vi "Acquire Connection.vi"(4 "error in (no error)":errorcluster, 7 "Connection String":string) -> (0 "error out":errorcluster, 2 "ADO Version":string, 3 "Connection":refnum<k7>)   [LabVIEW 2020, in "ADO Database Drivers.lvlib"]
uses:
  ADO Database Drivers.lvlib
panel:
  in  "?":refnum<k7>
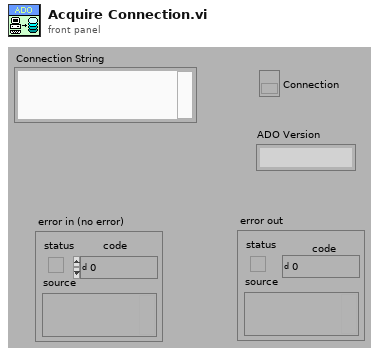
[diagram p1: front panel]
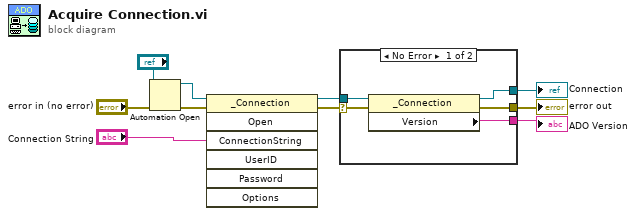
[diagram p0: block diagram]
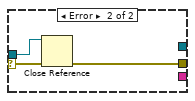
[diagram p2: hidden frame]
diagram:
  n1 = Automation Open(error in (no error)="error in (no error)", Automation Refnum="?") -> (Automation Refnum=w6:refnum<k7>, error out=w7:errorcluster)  [unwired: 2 in]
  n2 = invoke class="_Connection" method="Open"(reference=w6, error in=w7, "ConnectionString"="Connection String") -> (reference out=w4:refnum<k7>, error out=w5:errorcluster)  [unwired: 4 in, 5 out]
  n3 = case shown="No Error" w5 {
    selector: w5 -> [w15 w17]
    tunnel: w4 -> [w14 w18]
    tunnel: [w12 w16] -> w3
    tunnel: [w13 _] -> w2
    tunnel: [w11 _] -> w1
    frame No Error {
      n4 = property class="_Connection"(reference=w14, error in=w15) -> (reference out=w13:refnum<k7>, error out=w12:errorcluster, "Version"=w11:string)
    }
    frame Error {
      n5 = Close Reference(reference=w18, error in (no error)=w17) -> (error out=w16:errorcluster)
    }
  }
  "error out" <- w3
  "ADO Version" <- w1
  "Connection" <- w2
